vi "RestOperatingHoursEl.vi"(8 "Fehler (Eingang, kein Fehler)":errorcluster, 10 "DataFlowIN (Eingang)":T1, 11 "TableName":string) -> (0 "Fehler (Ausgang)":errorcluster, 2 "Calculeted Operating Hours":dbl, 3 "DataFlowIN (Ausgang)":T1)   [LabVIEW 2017]
uses:
  classes/DataCollector.lvclass
  classes/DataHandler.lvclass
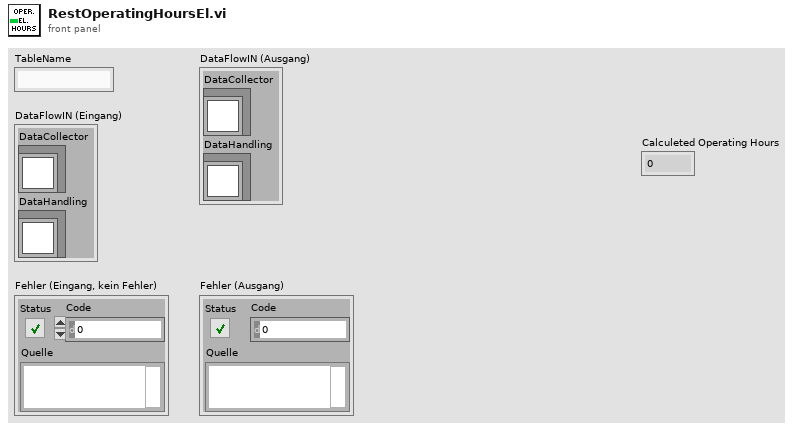
[diagram p1: front panel]
types:
  T1 = cluster{"DataCollector":refnum<class "DataCollector.lvclass">, "DataHandling":refnum<class "DataHandler.lvclass">}
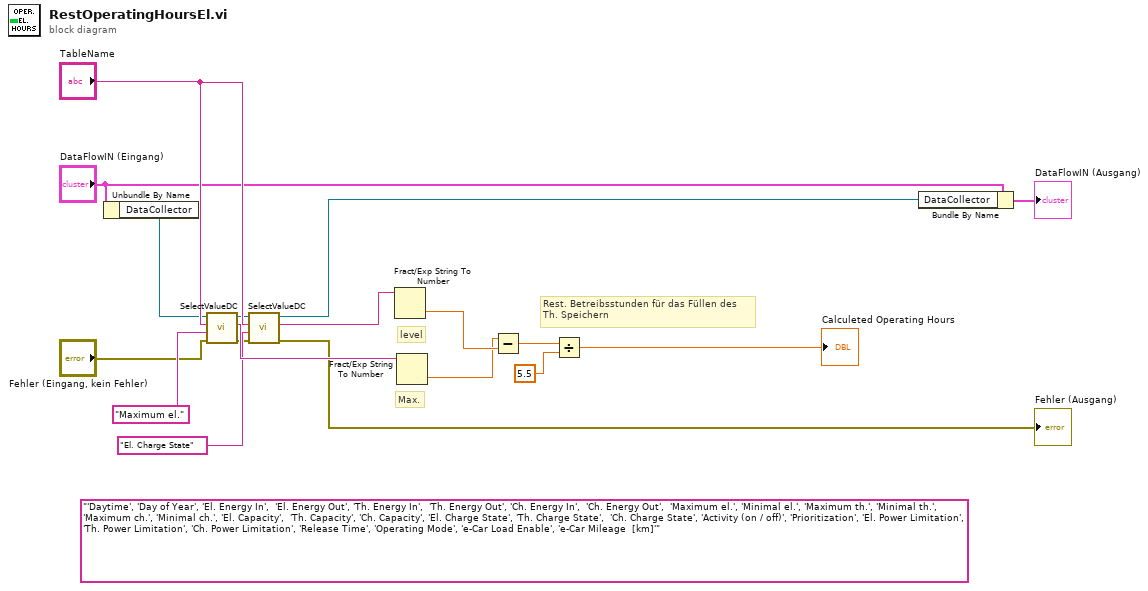
[diagram p0: block diagram]
diagram:
  (unwired) "'Daytime', 'Day of Year', 'El. Energy In',  'El. Energy Out', 'Th. Energy In',  'Th. Energy Out', 'Ch. Energy In',  'Ch. Energy Out',  'Maximum el.', 'Minimal el.', 'Maximum th.', 'Minimal th.',  'Maximum ch.', 'Minimal ch.', 'El. Capacity',  'Th. Capacity', 'Ch. Capacity', 'El. Charge State', 'Th. Charge State',  'Ch. Charge State', 'Activity (on / off)', 'Prioritization', 'El. Power Limitation',  'Th. Power Limitation', 'Ch. Power Limitation', 'Release Time', 'Operating Mode', 'e-Car Load Enable', 'e-Car Mileage  [km]'" ("string")
  # "Rest. Betreibsstunden für das Füllen des \nTh. Speichern"
  # "level"
  # "Max."
  n1 = Unbundle By Name("DataFlowIN (Eingang)") -> ("DataCollector"=w8:refnum<class "DataCollector.lvclass">)
  n2 = call-dynamic "SelectValueDC.vi"("error in (no error)"="Fehler (Eingang, kein Fehler)", "Table Row Name"="Maximum el.", "Unique Object Identifier"="TableName", "DataCollector in"=w8) -> ("error out"=w5:errorcluster, "Value"=w14:string, "DataCollector out"=w4:refnum<class "DataCollector.lvclass">)  [unwired: 5 in]
  n3 = call-dynamic "SelectValueDC.vi"("error in (no error)"=w5, "Table Row Name"="El. Charge State", "Unique Object Identifier"="TableName", "DataCollector in"=w4) -> ("error out"=→"Fehler (Ausgang)":errorcluster, "Value"=w13:string, "DataCollector out"=w12:refnum<class "DataCollector.lvclass">)  [unwired: 5 in]
  n4 = Fract/Exp String To Number(string=w13) -> (number=w16:dbl)  [unwired: 3 in, 1 out]
  n5 = Fract/Exp String To Number(string=w14) -> (number=w15:dbl)  [unwired: 3 in, 1 out]
  n6 = Subtract(x=w15, y=w16) -> (x-y=w17:dbl)
  n7 = Divide(x=w17, y=5.5) -> (x/y=→"Calculeted Operating Hours":dbl)
  n8 = Bundle By Name(cluster="DataFlowIN (Eingang)", "DataCollector"=w12) -> (→"DataFlowIN (Ausgang)":T1)
